vi "Alpha Ver 1.5.vi"() -> ()   [LabVIEW 2015]
uses:
  <instrlib>/Keithley 622x LV 2009/Configure/Source/Typedefs/KE622x -- Current Range.ctl
  <instrlib>/Keithley 622x LV 2009/Configure/Source/Typedefs/KE622x -- Current Ranges.ctl
  <instrlib>/Keithley 622x LV 2009/Typedefs/KE622x -- On Off Control.ctl
  <instrlib>/Keithley 622x LV 2009/Utility/Typedefs/KE622x -- Instrument Type.ctl
  <instrlib>/Keithley 622x LV 2009/Configure/Source/Typedefs/KE622x -- Voltage Limit.ctl
  <instrlib>/Keithley 2000/Public/Configure/Configure DC Volts.vi
  <userlib>/LV-Link3/PolySubVIs/DtCreateAinChan.vi
  <userlib>/LV-Link3/PolySubVIs/DtOLReadMultipleSingle.vi
  <instrlib>/Keithley 2000/Keithley 2000.lvlib
  <instrlib>/Keithley 622x LV 2009/Keithley 622x.lvlib
panel:
  in  "Setup":u16(ring) items=["START, STOP, STEP, CONFIGURATION", "PRINCETON LOCK-IN AMP"]
  out "prev_time_const":i32
  out "prev_range":i32
  out "XTC":i32
  out "SEN":i32
  in  "Time Delay":u16(ring) items=["0.1", "1", "3", "10", "30", "60"]
  out "FILE":refnum<file>
  out "Tick":u32
  in  "MULTIPLE GRAPHS Y":u16(ring) items=["Linear", "Log"]
  in  "MULTIPLE GRAPHS X":u16(ring) items=["Linear", "Log"]
  in  "TIME GRAPH Y":u16(ring) items=["Linear", "Log"]
  in  "TIME GRAPH X":u16(ring) items=["Linear", "Log"]
  in  "Lock-In, Y":dbl=1.0
  in  "Lock-In, X":dbl=1.0
  in  "DAQ A4":dbl=1.0
  in  "DAQ A3":dbl=1.0
  in  "DAQ A2":dbl=1.0
  in  "DAQ A1":dbl=1.0
  in  "DAQ A0":dbl=1.0
  in  "2000":dbl=1.0
  in  "Current":dbl=1000.0
  in  "Display Type 3":u16(ring)=3 items=["X %", "Y %", "X Calibrated", "Y Calibrated", "Mag %", "Mag Calibrated", "Phase Degrees", "Ratio", "ADC 1", "ADC 2", "ADC 3", "ADC 4 ", "Noise %", "Noise Calibrated", "Ref Frequency", "", ""]
  in  "Display Type 2":u16(ring)=2 items=["X %", "Y %", "X Calibrated", "Y Calibrated", "Mag %", "Mag Calibrated", "Phase Degrees", "Ratio", "ADC 1", "ADC 2", "ADC 3", "ADC 4 ", "Noise %", "Noise Calibrated", "Ref Frequency", "", ""]
  out "Units 3":string
  out "Display 3":dbl format="%.3f"
  out "Units 2":string
  out "Display 2":dbl format="%.3f"
  out "DAQ A4":dbl format="%#_13g"
  out "DAQ_clust":T1
  out "DAQ A3":dbl format="%#_13g"
  out "DAQ A2":dbl format="%#_13g"
  out "DAQ A1":dbl format="%#_13g"
  out "Real stop cur":dbl format="%#_13g"
  out "Real start cur":dbl format="%#_13g"
  in  "Stop cur prefix":u16(ring)=2
  in  "Start cur prefix":u16(ring)=2
  out "MULTIPLE GRAPHS":cluster{dbl[], dbl[]}[](graph)
  in  "X-Axis":T2(ring)
  in  "Range":u8(ring)=20 items=["100nV", "200nV", "500nV", "1µV", "2µV", "5µV", "10µV", "20µV", "50µV", "100µV", "200µV", "500µV", "1mV", "2mV", "5mV", "10mV", "20mV", "50mV", "100mV", "200mV", "500mV", "1V"]
  in  "Display Type copy":u16(ring)=3 items=["X %", "Y %", "X Calibrated", "Y Calibrated", "Mag %", "Mag Calibrated", "Phase Degrees", "Ratio", "ADC 1", "ADC 2", "ADC 3", "ADC 4 ", "Noise %", "Noise Calibrated", "Ref Frequency", "", ""]
  out "Units copy":string
  out "Display copy":dbl format="%.3f"
  out "Overload":bool
  out "Display":dbl format="%.3f"
  out "Units":string
  in  "Display Type":u16(ring)=2 items=["X %", "Y %", "X Calibrated", "Y Calibrated", "Mag %", "Mag Calibrated", "Phase Degrees", "Ratio", "ADC 1", "ADC 2", "ADC 3", "ADC 4 ", "Noise %", "Noise Calibrated", "Ref Frequency", "", ""]
  in  "Time Constant":u16(ring)=7 items=["MIN", "1ms", "3ms", "10ms", "30ms", "100ms", "300ms", "1s", "3s", "10s", "30s", "100s", "300s"]
  in  "Slope":u8(ring) items=["6db/octave", "12dB/octave"]
  in  "Dynamic Reserve":u16(ring)=1 items=["High Stability", "Normal", "High Reserve"]
  in  "Auto Sensitivity":bool
  in  "Auto Measure":bool
  out "6221_error_out":errorcluster
  out "2000_error_out":errorcluster
  out "5110_error_out":errorcluster
  out "Input Mode":i32(ring) items=[" Voltage Input (A or A-B) ", "Current Input 10E6 V/A", "Current Input 10E8 V/A"]
  out "5110":refnum<visa-resource-name>
  in  "GPIB Address":i8=11 min=1 max=32 step=1
  out "DAQ A0":dbl format="%#_13g"
  out "2000":dbl format="%#_13g"
  in  "Device":string(combo)
  in  "Number \nof points":i32=10
  in  "Folder\nprename":string
  out "TIME GRAPH":cluster{dbl[], dbl[]}[](graph)
  out "T0":u32
  out "LIMIT":bool
  out "LIMIT":bool
  out "Error Code":string
  in  "Comments":string
  out "2000":refnum<visa-resource-name>
  out "6221":refnum<visa-resource-name>
  out "Step  (A)":dbl=5e-05 format="%#_3p"
  in  "Stop\ncurrent (A)":dbl=2.0 format="%#_6p"
  in  "Start \ncurrent (A)":dbl=1.0 format="%#_6p"
  in  "Check For SCPI Errors? (T)":bool=TRUE
  out "Interlock Tripped?":bool
  out "Compliance?":bool
  in  "Turn Off Output \nIf Compliance?":bool=TRUE
  in  "Turning ON/OFF\ncurrent output":T3=enum."On"
  in  "Range Selection":T4={"Auto Range?"=TRUE, "Man / Selected\nRange"=enum."2nA"}
  # "FILE CONFIGURATION"
  # "ADMIN PANEL"
  # "MULTIPLIERS"
  # "SCALES"
  # "KEITHLEY 6221 CONFIGURATION (ADMIN ONLY)"
  # "KEITHLEY DAQ CONFIGURATION (ADMIN ONLY)"
  # "PRINCETON LOCK-IN AMP (ADMIN ONLY)"
  # "I don't know what the hell it is,\njust don't touch it"
  # "INPUT CONFIGURATION"
  # "READINGS"
  # "IF ON"
  # "Compliance = Limiting output voltage\nThis switch determines if we want to switch \noff the current output if wee exceed compliance"
  # "SCALES"
  # "There is a safe switch at \nthe back of the instrument \nThis indicator shows if it is on"
  # "You have hit a damn jackpot \nby exceeding the limited voltage\nCongrats"
  # "LOCK-IN READINGS"
  # "RIGHT DISPLAY"
  # "LEFT DISPLAY"
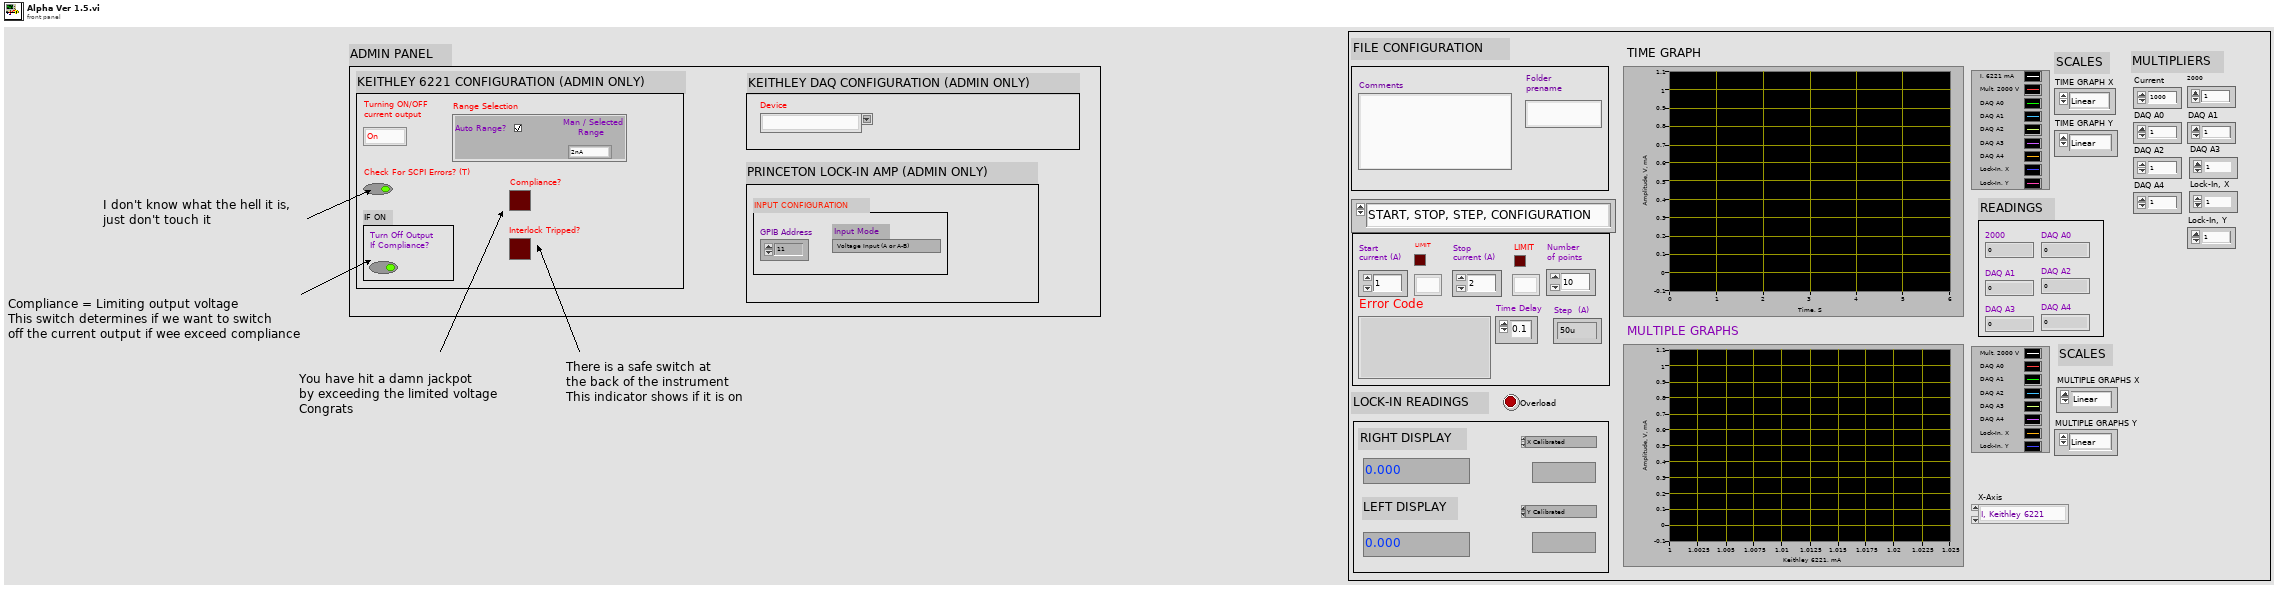
[diagram p1: front panel]
types:
  T1 = cluster{"Task out":i32, "Actual Number of Channels":u32, "error out":errorcluster}
  T2 = enum16{"I, Keithley 6221", "V, Keithley 2000", "V, Keithley DAQ A0", "V, Keithley DAQ A1", "V, Keithley DAQ A2", "V, Keithley DAQ A3", "V, Keithley DAQ A4", "V, Lock-In X", "V, Lock-In Y"}
  T3 = typedef "Keithley 622x.lvlib/KE622x -- On Off Control.ctl" = enum16{"Off", "On"}
  T4 = typedef "Keithley 622x.lvlib/KE622x -- Current Range.ctl" = cluster{"Auto Range?":bool, "Man / Selected\nRange":T5}
  T5 = typedef "Keithley 622x.lvlib/KE622x -- Current Ranges.ctl" = enum16{"2nA", "20nA", "200nA", "2uA", "20uA", "200uA", "2mA", "20mA", "100mA"}
  T6 = typedef "Keithley 622x.lvlib/KE622x -- Instrument Type.ctl" = enum16{"KE6220", "KE6221"}
  T7 = typedef "Keithley 622x.lvlib/KE622x -- Voltage Limit.ctl" = dbl
  T8 = cluster{"Task out":i32, "error out":errorcluster}
  T9 = cluster{dbl, dbl, dbl, dbl, dbl, "Measurement":dbl}
  T10 = cluster{dbl[], dbl[], dbl[], dbl[], dbl[], dbl[], dbl[], dbl[], dbl[], dbl[]}
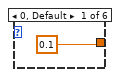
[diagram p2: hidden frame]
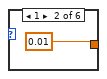
[diagram p3: hidden frame]
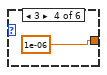
[diagram p4: hidden frame]
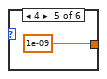
[diagram p5: hidden frame]
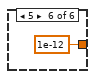
[diagram p6: hidden frame]
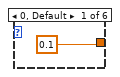
[diagram p7: hidden frame]
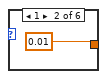
[diagram p8: hidden frame]
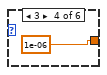
[diagram p9: hidden frame]
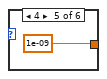
[diagram p10: hidden frame]
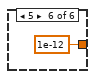
[diagram p11: hidden frame]
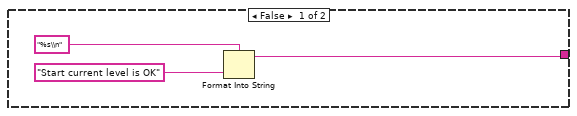
[diagram p12: hidden frame]
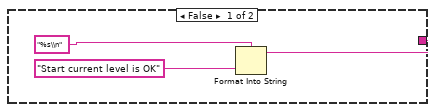
[diagram p13: hidden frame]
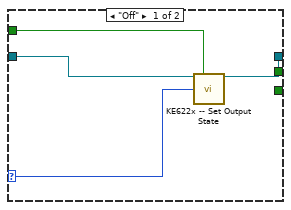
[diagram p14: hidden frame]
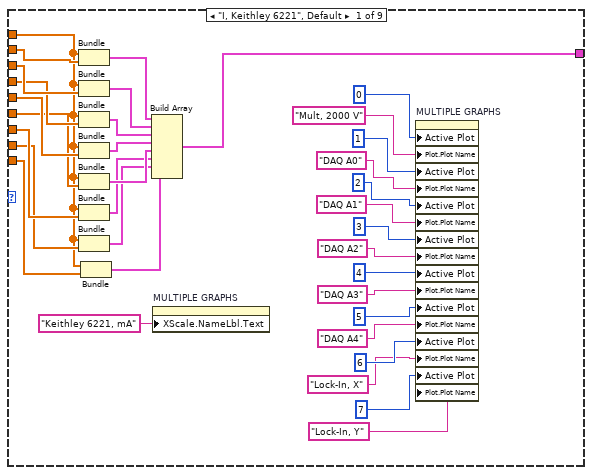
[diagram p15: hidden frame]
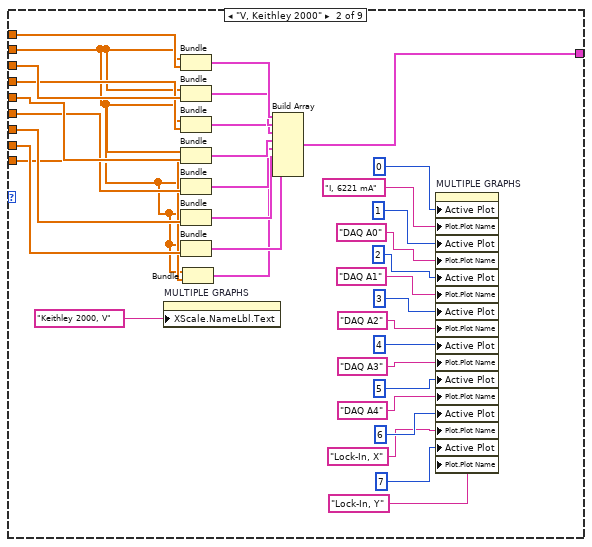
[diagram p16: hidden frame]
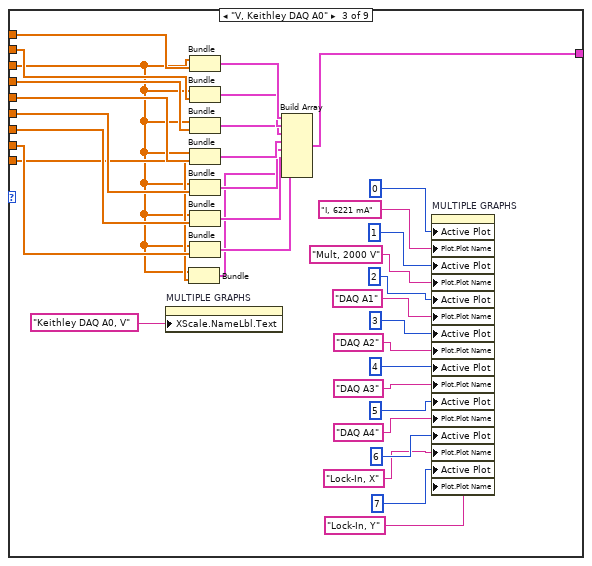
[diagram p17: hidden frame]
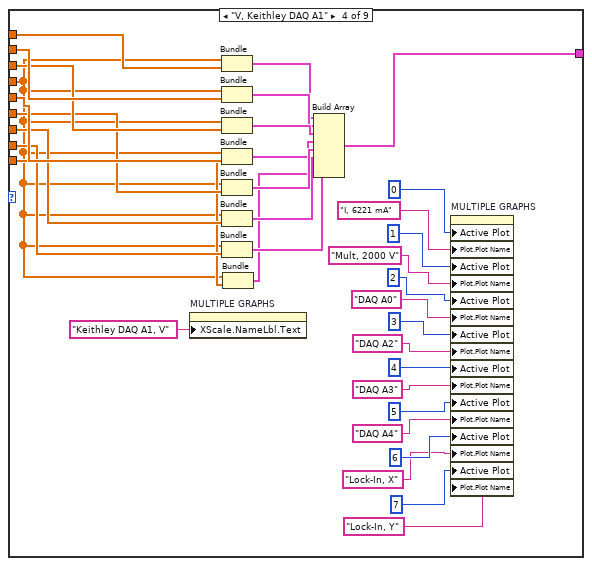
[diagram p18: hidden frame]
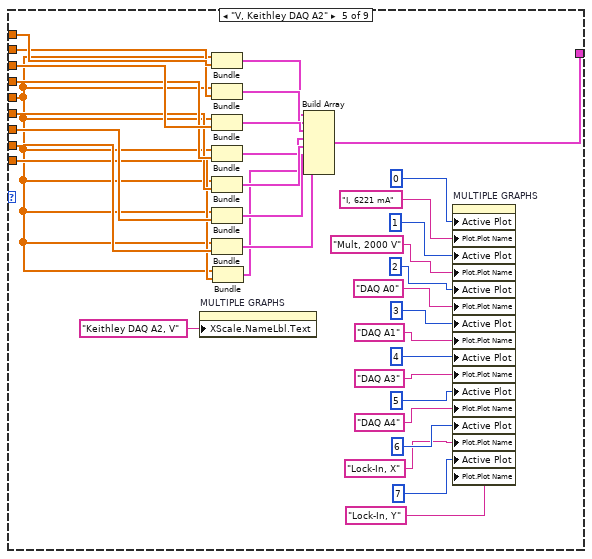
[diagram p19: hidden frame]
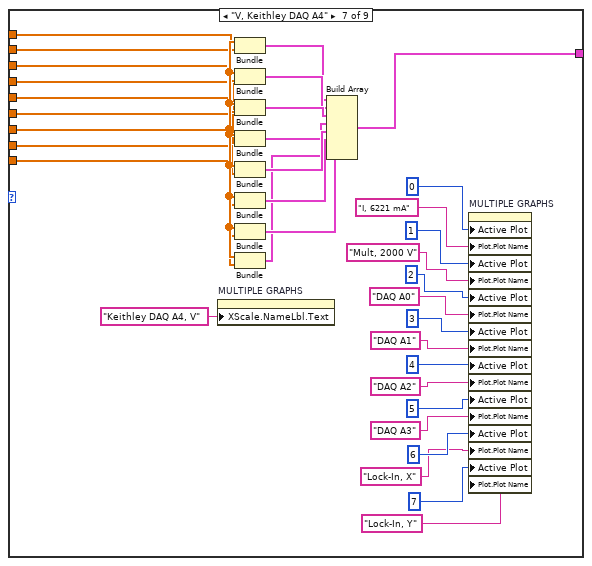
[diagram p20: hidden frame]
diagram:
  n1 = flat-sequence {
    tunnel: [w179] -> w7
    tunnel: [w178] -> w6
    tunnel: [w177] -> w5
    tunnel: [w176] -> w4
    tunnel: [w175] -> w3
    tunnel: [w174] -> w2
    tunnel: [w163] -> w1
    tunnel: w7 -> [w1126]
    tunnel: w6 -> [w1125]
    tunnel: w5 -> [w1124]
    tunnel: w4 -> [w1123]
    tunnel: w3 -> [w1122]
    tunnel: w2 -> [w1121]
    tunnel: w1 -> [w1120]
    frame #0 {
      # "File configuration"
      # "Start, Stop, Step"
      # "Initializing instruments"
      n2 = flat-sequence {
        frame #0 {
          w15 = TRUE  # reset
          w14 = FALSE  # ID query
          # "Initialize Lock-In 5110"
          # "Initialize Keithley 2000"
          # "Initialize Keithley 6221"
          n3 = call <instrlib>:"Initialize.vi"("VISA resource name"=refnum<visa-resource-name> "KEITHLEY_MULTIMETER") -> ("VISA resource name out"=w19:refnum<visa-resource-name>)  [unwired: 17 in, 1 out]
          n4 = call <instrlib>:"Initialize.vi"("VISA resource name"=refnum<visa-resource-name> "KEITHLEY_DC_AC_CURRENT_SOURCE", "Error Queue Option"=enum16{"Clear Error Queue", "Error Query"}."Clear Error Queue", "Instrument Type"=KE622x_--_Instrument_Type."KE6221") -> ("VISA resource name out"=→"6221":refnum<visa-resource-name>, "error out"=→"6221_error_out":errorcluster)  [unwired: 11 in]
          n5 = call "SR51XX Initialize"("VISA session (for class)"=refnum<visa-resource-name> "LOCK_IN_5110_PRINCETON", "Interface"=FALSE, "ID query"=w14, "GPIB Address"="GPIB Address", "reset"=w15) -> ("VISA session"=→"5110":refnum<visa-resource-name>, "error out"=→"5110_error_out":errorcluster)  [unwired: 8 in, 1 out]
          n6 = call-poly <instrlib>:"Configure Measurement.vi"("VISA resource name"=w19) -> ("VISA resource name out"=→"2000":refnum<visa-resource-name>, "error out"=→"2000_error_out":errorcluster)  [unwired: 17 in]
        }
        frame #1 {
          # "Initialize Keithley DAQ \n(getting board name)"
          n7 = call <userlib>:"DtOLGetBoardNames.vi"() -> ("Number of boards"=w24:u32)  [unwired: 9 in, 2 out]
          n8 = Initialize Array("", w24) -> (w26:string[])
          n9 = for {
            N: w24 -> [_]
            shift-right: [w32] -> w29
            shift-left: w26 -> [w33]
            i -> [w31]
            n10 = Add(x=1, y=w31) -> (x+y=w35:i32)
            n11 = call <userlib>:"DtOLGetBoardNames.vi"("Select Board"=w35) -> ("Board Name"=w30:string)  [unwired: 8 in, 2 out]
            n12 = Replace Array Subset(array=w33, new element=w30, index=w31) -> (w32:string[])
          }
          n13 = Index Array(array=w29, index=0) -> (element=w28:string)
          n14 = property on="Device" class="CmbBox"("Strings[]"=w29, "Value"=w28) -> ()  [unwired: 2 in, 2 out]
        }
        frame #2 {
          # "Calculating steps by number\nof points"
          # "Putting in a loop \ninstead of \"STOP\""
          n15 = local read "Real stop cur"() -> (w52:dbl)
          n16 = local read "Real start cur"() -> (w53:dbl)
          n17 = case shown="2" "Start cur prefix" {
            tunnel: [0.1 0.01 0.001 1e-06 1e-09 1e-12] -> w41
            frame 0, Default {
            }
            frame 1 {
            }
            frame 2 {
            }
            frame 3 {
            }
            frame 4 {
            }
            frame 5 {
            }
          }
          n18 = case shown="2" "Stop cur prefix" {
            tunnel: [0.1 0.01 0.001 1e-06 1e-09 1e-12] -> w39
            frame 0, Default {
            }
            frame 1 {
            }
            frame 2 {
            }
            frame 3 {
            }
            frame 4 {
            }
            frame 5 {
            }
          }
          n19 = Subtract(x=w52, y=w53) -> (x-y=w55:dbl)
          n20 = Multiply(x=w41, y="Start \ncurrent (A)") -> (x*y=w37:dbl)
          "Real start cur" <- w37
          n21 = Divide(x=w55, y="Number \nof points") -> (x/y=→"Step  (A)":dbl)
          n22 = Multiply(x=w39, y="Stop\ncurrent (A)") -> (x*y=w36:dbl)
          "Real stop cur" <- w36
          n23 = Greater?(x=w36, y=T7 0.01) -> (0:w47:bool)
          n24 = Greater?(x=w37, y=T7 0.01) -> (0:w46:bool)
          n25 = case shown="True" w47 {
            selector: w47 -> [_ w71]
            tunnel: [w68 w74] -> w49
            frame False {
              n26 = Format Into String(format string="%s\\n", "Start current level is OK" ("false string")) -> (resulting string=w68:string)  [unwired: 2 in, 1 out]
            }
            frame True {
              n27 = flat-sequence {
                tunnel: [w76] -> w73
                tunnel: [w75] -> w72
                tunnel: w71 -> [w75]
                tunnel: [w80] -> w74
                tunnel: w73 -> [w80]
                tunnel: w72 -> [w81]
                frame #0 {
                  n28 = Format Into String(format string="%s\\n%s\\n", "Stop current level" ("String"), "exceeded the  limit: 10mA" ("input 2")) -> (resulting string=w76:string)  [unwired: 2 in, 1 out]
                }
                frame #1 {
                  n29 = while {
                    tunnel: w81 -> [w82]
                    stop <- w82 continue-if-true
                    "LIMIT" <- w82
                  }
                  n30 = property on="Error Code" class="Str"("Text.Text"=w80) -> ()  [unwired: 2 in, 2 out]
                }
              }
            }
          }
          n31 = case shown="True" w46 {
            selector: w46 -> [_ w87]
            tunnel: [w83 w89] -> w48
            frame False {
              n32 = Format Into String(format string="%s\\n", "Start current level is OK" ("false string")) -> (resulting string=w83:string)  [unwired: 2 in, 1 out]
            }
            frame True {
              n33 = flat-sequence {
                tunnel: [w91] -> w88
                tunnel: w87 -> [w90]
                tunnel: [w90] -> w86
                tunnel: [w95] -> w89
                tunnel: w88 -> [w95]
                tunnel: w86 -> [w96]
                frame #0 {
                  n34 = Format Into String(format string="%s\\n%s\\n", "Start current level" ("String"), "exceeded the limit: 10mA" ("input 2")) -> (resulting string=w91:string)  [unwired: 2 in, 1 out]
                }
                frame #1 {
                  n35 = while {
                    tunnel: w96 -> [w97]
                    stop <- w97 continue-if-true
                    "LIMIT" <- w97
                  }
                  n36 = property on="Error Code" class="Str"("Text.Text"=w95) -> ()  [unwired: 2 in, 2 out]
                }
              }
            }
          }
          n37 = Concatenate Strings(w48, w49) -> (→"Error Code":string)
        }
        frame #3 {
          # "Adding headlines"
          # "Creating folder&file"
          # "Creating comments"
          # "Writing instr params"
          n38 = local read "5110"() -> (w110:refnum<visa-resource-name>)
          n39 = local read "Real stop cur"() -> (w112:dbl)
          n40 = local read "Real start cur"() -> (w111:dbl)
          n41 = call "folder_creation.vi"("Name"="Folder\nprename") -> ("String"=w119:string)
          n42 = call "file_creation.vi"("String"=w119) -> ("refnum out"=w113:refnum<file>)
          "FILE" <- w113
          n43 = call "com_inst.vi"("Stop current"=w112, "Start current"=w111, "VISA session (for class)"=w110) -> ("XTC"=w108:i32, "SEN"=w109:i32, "concatenated string"=w107:string)
          "SEN" <- w109
          "XTC" <- w108
          n44 = Format Into String(format string="# %s\\n", initial string=w113, "Comments") -> (resulting string=w115:refnum<file>)  [unwired: 1 in, 1 out]
          n45 = property on="Time Constant" class="Ring (strict)"("Value"=w108) -> ()  [unwired: 2 in, 2 out]
          n46 = Format Into String(format string="# %s\\n", initial string=w115, w107) -> (resulting string=w114:refnum<file>)  [unwired: 1 in, 1 out]
          n47 = property on="Range" class="Ring (strict)"("Value"=w109) -> ()  [unwired: 2 in, 2 out]
          n48 = Format Into String(format string="# %-6s  %-12s %-12s %-14s %-12s %-14s %-12s %-12s %-14s%-14s\\n", initial string=w114, "t, ms" ("input 3"), "6221, A" ("input 3"), "2000, V" ("input 1"), "5110_X, V" ("input 3"), "5110_Y, V " ("input 3"), "DAQ A0, V" ("input 2"), "DAQ A1, V" ("input 2"), "DAQ A2, V" ("input 2"), "DAQ A3, V" ("input 2"), "DAQ A4, V" ("input 2")) -> ()  [unwired: 1 in, 2 out]
        }
        frame #4 {
          # "Variables"
          # "Time Intit"
          n49 = property on="SEN" class="DigNum (strict)"() -> ("Value"=→"prev_range":i32)  [unwired: 2 in, 2 out]
          n50 = property on="XTC" class="DigNum (strict)"() -> ("Value"=→"prev_time_const":i32)  [unwired: 2 in, 2 out]
          n51 = Wait Until Next ms Multiple(millisecond multiple=u32 1000) -> (millisecond timer value=→"T0":u32)
        }
      }
    }
    frame #1 {
      # "Configuring Keithley DAQ just before measuments"
      # "Configuring Keithley 6221 just before measuments"
      n52 = flat-sequence {
        tunnel: [w137] -> w127
        tunnel: [w155] -> _
        tunnel: [w157] -> _
        tunnel: w127 -> [w156]
        frame #0 {
          # "Current range \nselection check"
          # "Checking for compliance\nand interlock errors"
          n53 = local read "6221"() -> (w140:refnum<visa-resource-name>)
          n54 = call <instrlib>:"KE622x -- Set Current Range.vi"("Resource In"=w140, "Current Range In"="Range Selection", "Read Back Set Values? (T)"=FALSE) -> ("Resource Out (dupl)"=w145:refnum<visa-resource-name>)  [unwired: 10 in, 2 out]
          n55 = case shown="\"On\"" "Turning ON/OFF\ncurrent output" {
            selector: "Turning ON/OFF\ncurrent output" -> [w149 _]
            tunnel: [_ w153] -> w143
            tunnel: [_ w152] -> w144
            tunnel: "Check For SCPI Errors? (T)" -> [w148 _]
            tunnel: w145 -> [w146 w151]
            tunnel: [w147 w150] -> w137
            frame "Off" {
              n56 = call <instrlib>:"KE622x -- Set Output State.vi"("Resource In"=w146, "Check For SCPI Errors? (T)"=w148, "Output State"=w149) -> ("Resource Out (dupl)"=w147:refnum<visa-resource-name>)  [unwired: 11 in, 1 out]
            }
            frame "On" {
              n57 = call <instrlib>:"KE622x -- Turn Output On And Check For Errors.vi"("Resource In"=w151, "Turn Off Output If Compliance?"="Turn Off Output \nIf Compliance?") -> ("Resource Out (dupl)"=w150:refnum<visa-resource-name>, "Interlock Tripped?"=w153:bool, "Compliance?"=w152:bool)  [unwired: 10 in, 1 out]
            }
          }
          "Interlock Tripped?" <- w143
          "Compliance?" <- w144
        }
        frame #1 {
          # "Setting start current"
          n58 = local read "Real start cur"() -> (w155:dbl)
          n59 = Wait (ms)(milliseconds to wait=u32 100) -> ()  [unwired: 1 out]
          n60 = call <instrlib>:"KE622x -- Set Current Level.vi"("Resource In"=w156, "Current Level (A) In"=w155) -> ("Resource Out (dupl)"=w157:refnum<visa-resource-name>)  [unwired: 12 in, 1 out]
        }
      }
      n61 = flat-sequence {
        frame #0 {
          w132 = 100 items=["SingleEnded"=100, "Differential"=101] ("Channel Type")
          # "Configure the input channel"
          n62 = call-poly <userlib>:"DtOLCreateTask.vi"("Channel Type"=w132, "Range Min"=-10.0, "Range Max"=10.0, "Board Name"="Device", "Channel"="0:4" ("Channels")) -> ("Task out"=w131:i32, "Actual Number of Channels"=w130:u32, "error out"=w129:errorcluster)  [unwired: 8 in]
          n63 = Bundle("Task out"=w131, "Actual Number of Channels"=w130, "error out"=w129) -> (→"DAQ_clust":T1)  [unwired: 1 in]
        }
      }
    }
    frame #2 {
      n64 = local read "5110"() -> (w170:refnum<visa-resource-name>)
      n65 = local read "2000"() -> (w169:refnum<visa-resource-name>)
      n66 = local read "6221"() -> (w168:refnum<visa-resource-name>)
      n67 = local read "5110_error_out"() -> (w167:errorcluster)
      n68 = local read "6221_error_out"() -> (w166:errorcluster)
      n69 = local read "2000_error_out"() -> (w165:errorcluster)
      n70 = local read "DAQ_clust"() -> (w164:T1)
      n71 = while {
        shift-right: [w380] -> _
        shift-left: dbl[] [] -> [w481]
        shift-right: [w381] -> _
        shift-left: i32[] [] -> [w480]
        tunnel: w169 -> [w478]
        tunnel: w168 -> [w477]
        shift-right: [w338] -> _
        shift-left: dbl[] [] -> [w471]
        tunnel: [w470] -> w179
        tunnel: [w469] -> w178
        tunnel: [w467] -> w177
        tunnel: [w465] -> w176
        tunnel: w170 -> [w463]
        tunnel: w167 -> [w462]
        tunnel: w166 -> [w454]
        tunnel: w165 -> [w453]
        tunnel: [w428] -> w175
        tunnel: [w426] -> w174
        shift-right: [w340] -> _
        shift-left: dbl[] [] -> [w425]
        shift-right: [w341] -> _
        shift-left: dbl[] [] -> [w424]
        shift-right: [w382] -> _
        shift-left: dbl[] [] -> [w421]
        tunnel: w164 -> [w395]
        tunnel: [w394] -> w163
        shift-right: [w379] -> _
        shift-left: dbl[] [] -> [w393]
        shift-right: [w378] -> _
        shift-left: dbl[] [] -> [w392]
        shift-right: [w377] -> _
        shift-left: dbl[] [] -> [w391]
        shift-right: [w339] -> _
        shift-left: dbl[] [] -> [w343]
        i -> [w455]
        stop <- w472 stop-if-true
        # "V, DAQ A4"
        # "V, DAQ A3"
        # "V, DAQ A2"
        # "V, DAQ A1"
        # "Y-V, 5110"
        # "X-V, 5110"
        # "I, 6221"
        # "Config delay"
        # "Control subVI 5110"
        # "Read config 5110"
        # "Measurement config 5110"
        # "Time config 5110"
        # "Configuring Right Display 5110"
        # "Configuring Left Display 5110"
        # "Setting 6221 current"
        # "Delay before measuremens"
        # "Getting the data from DAQ and 2000"
        # "Changing input current"
        # "Time"
        # "V, DAQ A0"
        # "V, 2000"
        n72 = local read "T0"() -> (w479:u32)
        n73 = Quotient & Remainder(x=w455, y=10) -> (floor(x/y)=w460:i32)  [unwired: 1 out]
        n74 = Equal?(x=0, y=w455) -> (x = y?=w457:bool)
        n75 = Subtract(x=w446, y=w479) -> (x-y=w402:u32)
        n76 = Equal?(x=1, y=w460) -> (x = y?=w456:bool)
        n77 = flat-sequence {
          tunnel: w478 -> [w806]
          tunnel: [w806] -> w420
          tunnel: w477 -> [w805]
          tunnel: [w805] -> w418
          tunnel: w463 -> [w804]
          tunnel: [w804] -> w416
          tunnel: [w803] -> w414
          tunnel: w462 -> [w803]
          tunnel: w457 -> [w802]
          tunnel: [w802] -> w412
          tunnel: w456 -> [w801]
          tunnel: [w801] -> w410
          tunnel: w454 -> [w800]
          tunnel: [w800] -> w408
          tunnel: w453 -> [w799]
          tunnel: [w799] -> w406
          tunnel: [w797] -> w446
          tunnel: [w798] -> w396
          tunnel: w395 -> [w798]
          tunnel: w420 -> [w816]
          tunnel: [w816] -> w419
          tunnel: w418 -> [w815]
          tunnel: [w815] -> w417
          tunnel: w416 -> [w814]
          tunnel: [w814] -> w415
          tunnel: w414 -> [w813]
          tunnel: [w813] -> w413
          tunnel: w412 -> [w812]
          tunnel: [w812] -> w411
          tunnel: w410 -> [w811]
          tunnel: [w811] -> w409
          tunnel: w408 -> [w810]
          tunnel: [w810] -> w407
          tunnel: w406 -> [w809]
          tunnel: [w809] -> w405
          tunnel: [w808] -> w397
          tunnel: w396 -> [w808]
          tunnel: w419 -> [w861]
          tunnel: [w861] -> w445
          tunnel: w417 -> [w860]
          tunnel: [w860] -> w444
          tunnel: w415 -> [w859]
          tunnel: w413 -> [w856]
          tunnel: [w855] -> w443
          tunnel: [w854] -> w442
          tunnel: w411 -> [w853]
          tunnel: [w853] -> w441
          tunnel: w409 -> [w852]
          tunnel: w407 -> [w851]
          tunnel: [w851] -> w440
          tunnel: w405 -> [w850]
          tunnel: [w850] -> w439
          tunnel: [w849] -> w398
          tunnel: w397 -> [w849]
          tunnel: w445 -> [w886]
          tunnel: [w886] -> w239
          tunnel: w444 -> [w885]
          tunnel: [w885] -> w237
          tunnel: w443 -> [w882]
          tunnel: [w881] -> w235
          tunnel: w442 -> [w880]
          tunnel: [w879] -> w233
          tunnel: w441 -> [w877]
          tunnel: [w877] -> w231
          tunnel: w440 -> [w884]
          tunnel: [w884] -> w229
          tunnel: w439 -> [w883]
          tunnel: [w883] -> w227
          tunnel: ["Auto Measure"] -> w225
          tunnel: ["Auto Sensitivity"] -> w223
          tunnel: [w872] -> w221
          tunnel: [w870] -> w219
          tunnel: w398 -> [w870]
          tunnel: w239 -> [w900]
          tunnel: [w900] -> w238
          tunnel: w237 -> [w899]
          tunnel: [w899] -> w236
          tunnel: w235 -> [w887]
          tunnel: [w887] -> w234
          tunnel: w233 -> [w898]
          tunnel: [w898] -> w232
          tunnel: w231 -> [w897]
          tunnel: [w897] -> w230
          tunnel: w229 -> [w896]
          tunnel: [w896] -> w228
          tunnel: w227 -> [w895]
          tunnel: [w895] -> w226
          tunnel: w225 -> [w894]
          tunnel: [w894] -> w224
          tunnel: w223 -> [w893]
          tunnel: [w893] -> w222
          tunnel: w221 -> [w892]
          tunnel: [w892] -> w220
          tunnel: w219 -> [w891]
          tunnel: [w891] -> w218
          tunnel: w238 -> [w927]
          tunnel: [w927] -> w195
          tunnel: w236 -> [w926]
          tunnel: [w926] -> w197
          tunnel: w234 -> [w919]
          tunnel: w232 -> [w917]
          tunnel: [w916] -> w199
          tunnel: w230 -> [w923]
          tunnel: [w923] -> w201
          tunnel: w228 -> [w925]
          tunnel: [w925] -> w203
          tunnel: w226 -> [w924]
          tunnel: [w924] -> w205
          tunnel: w224 -> [w921]
          tunnel: [w921] -> w207
          tunnel: w222 -> [w922]
          tunnel: [w922] -> w209
          tunnel: w220 -> [w912]
          tunnel: [w912] -> w211
          tunnel: [w918] -> w213
          tunnel: ["Time Constant"] -> w215
          tunnel: ["Slope"] -> w217
          tunnel: [w910] -> w193
          tunnel: w218 -> [w910]
          tunnel: w217 -> [w943]
          tunnel: [w943] -> w216
          tunnel: w215 -> [w942]
          tunnel: [w942] -> w214
          tunnel: w213 -> [w930]
          tunnel: [w930] -> w212
          tunnel: w211 -> [w941]
          tunnel: [w941] -> w210
          tunnel: w209 -> [w940]
          tunnel: [w940] -> w208
          tunnel: w207 -> [w939]
          tunnel: [w939] -> w206
          tunnel: w205 -> [w938]
          tunnel: [w938] -> w204
          tunnel: w203 -> [w937]
          tunnel: [w937] -> w202
          tunnel: w201 -> [w936]
          tunnel: [w936] -> w200
          tunnel: w199 -> [w932]
          tunnel: [w932] -> w198
          tunnel: w197 -> [w935]
          tunnel: [w935] -> w196
          tunnel: w195 -> [w934]
          tunnel: [w934] -> w194
          tunnel: w193 -> [w933]
          tunnel: [w933] -> w192
          tunnel: [w973] -> w336
          tunnel: [w972] -> w335
          tunnel: [w958] -> w334
          tunnel: [w971] -> w333
          tunnel: [w970] -> w332
          tunnel: [w969] -> w331
          tunnel: [w968] -> w330
          tunnel: [w967] -> w329
          tunnel: [w960] -> w328
          tunnel: [w963] -> w327
          tunnel: [w961] -> w326
          tunnel: [w966] -> w325
          tunnel: w216 -> [w966]
          tunnel: w214 -> [w961]
          tunnel: w212 -> [w964]
          tunnel: w210 -> [w960]
          tunnel: w208 -> [w967]
          tunnel: w206 -> [w968]
          tunnel: w204 -> [w969]
          tunnel: w202 -> [w970]
          tunnel: w200 -> [w971]
          tunnel: w198 -> [w959]
          tunnel: w196 -> [w972]
          tunnel: w194 -> [w973]
          tunnel: [w952] -> w324
          tunnel: w192 -> [w952]
          tunnel: w336 -> [w996]
          tunnel: [w996] -> w323
          tunnel: w335 -> [w995]
          tunnel: [w995] -> w321
          tunnel: w334 -> [w987]
          tunnel: [w986] -> w319
          tunnel: w333 -> [w994]
          tunnel: [w994] -> w317
          tunnel: w332 -> [w993]
          tunnel: [w993] -> w315
          tunnel: w331 -> [w992]
          tunnel: [w992] -> w313
          tunnel: w330 -> [w991]
          tunnel: [w991] -> w311
          tunnel: w329 -> [w990]
          tunnel: [w990] -> w309
          tunnel: w328 -> [w981]
          tunnel: [w981] -> w307
          tunnel: w327 -> [w988]
          tunnel: [w985] -> w305
          tunnel: w326 -> [w983]
          tunnel: [w983] -> w303
          tunnel: w325 -> [w980]
          tunnel: [w980] -> w301
          tunnel: w324 -> [w989]
          tunnel: [w989] -> w299
          tunnel: [w976] -> w296
          tunnel: w323 -> [w1019]
          tunnel: [w1019] -> w322
          tunnel: w321 -> [w1018]
          tunnel: [w1018] -> w320
          tunnel: w319 -> [w1009]
          tunnel: [w1008] -> w318
          tunnel: w317 -> [w1017]
          tunnel: [w1017] -> w316
          tunnel: w315 -> [w1016]
          tunnel: [w1016] -> w314
          tunnel: w313 -> [w1015]
          tunnel: [w1015] -> w312
          tunnel: w311 -> [w1014]
          tunnel: [w1014] -> w310
          tunnel: w309 -> [w1013]
          tunnel: [w1013] -> w308
          tunnel: w307 -> [w1004]
          tunnel: [w1004] -> w306
          tunnel: w305 -> [w1011]
          tunnel: [w1010] -> w304
          tunnel: w303 -> [w1006]
          tunnel: [w1006] -> w302
          tunnel: w301 -> [w1003]
          tunnel: [w1003] -> w300
          tunnel: w299 -> [w1012]
          tunnel: [w1012] -> w298
          tunnel: [w999] -> w297
          tunnel: w322 -> [w1041]
          tunnel: [w1041] -> w438
          tunnel: w320 -> [w1040]
          tunnel: [w1040] -> w437
          tunnel: w318 -> [w1027]
          tunnel: w316 -> [w1039]
          tunnel: [w1039] -> w436
          tunnel: w314 -> [w1038]
          tunnel: [w1038] -> w435
          tunnel: w312 -> [w1037]
          tunnel: [w1037] -> w434
          tunnel: w310 -> [w1036]
          tunnel: [w1036] -> w433
          tunnel: w308 -> [w1035]
          tunnel: [w1035] -> w432
          tunnel: w306 -> [w1028]
          tunnel: w304 -> [w1025]
          tunnel: [w1024] -> w431
          tunnel: w302 -> [w1029]
          tunnel: w300 -> [w1030]
          tunnel: [w1026] -> w430
          tunnel: [w1023] -> w429
          tunnel: [w1020] -> w399
          tunnel: w298 -> [w1020]
          tunnel: [w1045] -> w476
          tunnel: w455 -> [w1053]
          tunnel: [w1049] -> w472
          tunnel: [w1043] -> w474
          tunnel: [w1051] -> w473
          tunnel: [w1048] -> w452
          tunnel: [w1047] -> w451
          tunnel: [w1046] -> w450
          tunnel: [w1044] -> w449
          tunnel: [w1043] -> w390
          tunnel: w429 -> [_]
          tunnel: w430 -> [w1046]
          tunnel: w431 -> [w1044]
          tunnel: w432 -> [_]
          tunnel: w433 -> [_]
          tunnel: w434 -> [w1048]
          tunnel: w435 -> [w1047]
          tunnel: w436 -> [_]
          tunnel: w437 -> [w1051]
          tunnel: w438 -> [w1045]
          tunnel: [w1042] -> w400
          tunnel: w399 -> [w1042]
          tunnel: w476 -> [w1066]
          tunnel: [w1066] -> w475
          tunnel: w474 -> [w1065]
          tunnel: w473 -> [w1064]
          tunnel: [w1063] -> w468
          tunnel: [w1062] -> w466
          tunnel: w452 -> [w1060]
          tunnel: w451 -> [w1061]
          tunnel: w450 -> [w1058]
          tunnel: w449 -> [w1059]
          tunnel: [w1060] -> w448
          tunnel: [w1059] -> w447
          tunnel: [w1058] -> w427
          tunnel: [w1057] -> w401
          tunnel: w400 -> [w1057]
          tunnel: [w1103] -> w365
          tunnel: [w1070] -> w364
          tunnel: [w1102] -> w363
          tunnel: [w1101] -> w362
          tunnel: [w1100] -> w361
          tunnel: [w1099] -> w360
          tunnel: [w1071] -> w359
          tunnel: [w1103] -> w358
          tunnel: [w1098] -> w357
          tunnel: [w1097] -> w356
          tunnel: [w1096] -> w355
          tunnel: [w1069] -> w354
          tunnel: [w1068] -> w353
          tunnel: [w1067] -> w352
          tunnel: w401 -> [w1093]
          tunnel: w427 -> [w1097]
          tunnel: w447 -> [w1098]
          tunnel: w448 -> [w1094]
          tunnel: w466 -> [w1099]
          tunnel: w468 -> [w1100]
          tunnel: w475 -> [w1095]
          tunnel: [w1107] -> w394
          tunnel: [w1108] -> w426
          tunnel: [w1109] -> w428
          tunnel: [w1110] -> w464
          tunnel: [w1111] -> w351
          tunnel: [w1112] -> w465
          tunnel: [w1113] -> w467
          tunnel: [w1114] -> w469
          tunnel: [w1115] -> w470
          tunnel: [w1116] -> w350
          tunnel: [w1117] -> w346
          tunnel: w365 -> [w1117]
          tunnel: w364 -> [w1116]
          tunnel: w363 -> [w1115]
          tunnel: w362 -> [w1114]
          tunnel: w361 -> [w1113]
          tunnel: w360 -> [w1112]
          tunnel: w359 -> [w1111]
          tunnel: w358 -> [w1110]
          tunnel: w357 -> [w1109]
          tunnel: w356 -> [w1108]
          tunnel: w355 -> [w1107]
          tunnel: [w1106] -> w349
          tunnel: w354 -> [w1106]
          tunnel: [w1105] -> w348
          tunnel: w353 -> [w1105]
          tunnel: w352 -> [w1104]
          tunnel: [w1104] -> w347
          frame #0 {
            n78 = Tick Count (ms)() -> (millisecond timer value=w797:u32)
            "Tick" <- w797
          }
          frame #1 {
            n79 = case shown="0, Default" "Setup" {
              frame 0, Default {
                n80 = property on="Slope" class="Ring (strict)"("Visible"=FALSE) -> ()  [unwired: 2 in, 2 out]
                n81 = property on="Start \ncurrent (A)" class="DigNum (strict)"("Visible"=TRUE) -> ()  [unwired: 2 in, 2 out]
                n82 = property on="LIMIT" class="Bool (strict)"("Visible"=TRUE) -> ()  [unwired: 2 in, 2 out]
                n83 = property on="Start cur prefix" class="Ring (strict)"("Visible"=TRUE) -> ()  [unwired: 2 in, 2 out]
                n84 = property on="Step  (A)" class="DigNum (strict)"("Visible"=TRUE) -> ()  [unwired: 2 in, 2 out]
                n85 = property on="Dynamic Reserve" class="Ring (strict)"("Visible"=FALSE) -> ()  [unwired: 2 in, 2 out]
                n86 = property on="Range" class="Ring (strict)"("Visible"=FALSE) -> ()  [unwired: 2 in, 2 out]
                n87 = property on="LIMIT" class="Bool (strict)"("Visible"=TRUE) -> ()  [unwired: 2 in, 2 out]
                n88 = property on="Stop\ncurrent (A)" class="DigNum (strict)"("Visible"=TRUE) -> ()  [unwired: 2 in, 2 out]
                n89 = property on="Stop cur prefix" class="Ring (strict)"("Visible"=TRUE) -> ()  [unwired: 2 in, 2 out]
                n90 = property on="Time Delay" class="Ring (strict)"("Visible"=TRUE) -> ()  [unwired: 2 in, 2 out]
                n91 = property on="Auto Sensitivity" class="Bool (strict)"("Visible"=FALSE) -> ()  [unwired: 2 in, 2 out]
                n92 = property on="Time Constant" class="Ring (strict)"("Visible"=FALSE) -> ()  [unwired: 2 in, 2 out]
                n93 = property on="Number \nof points" class="DigNum (strict)"("Visible"=TRUE) -> ()  [unwired: 2 in, 2 out]
                n94 = property on="Auto Measure" class="Bool (strict)"("Visible"=FALSE) -> ()  [unwired: 2 in, 2 out]
                n95 = property on="Error Code" class="Str"("Visible"=TRUE) -> ()  [unwired: 2 in, 2 out]
              }
              frame 1 {
                n96 = property on="Slope" class="Ring (strict)"("Visible"=TRUE) -> ()  [unwired: 2 in, 2 out]
                n97 = property on="Start \ncurrent (A)" class="DigNum (strict)"("Visible"=FALSE) -> ()  [unwired: 2 in, 2 out]
                n98 = property on="LIMIT" class="Bool (strict)"("Visible"=FALSE) -> ()  [unwired: 2 in, 2 out]
                n99 = property on="Start cur prefix" class="Ring (strict)"("Visible"=FALSE) -> ()  [unwired: 2 in, 2 out]
                n100 = property on="Step  (A)" class="DigNum (strict)"("Visible"=FALSE) -> ()  [unwired: 2 in, 2 out]
                n101 = property on="Dynamic Reserve" class="Ring (strict)"("Visible"=TRUE) -> ()  [unwired: 2 in, 2 out]
                n102 = property on="Range" class="Ring (strict)"("Visible"=TRUE) -> ()  [unwired: 2 in, 2 out]
                n103 = property on="LIMIT" class="Bool (strict)"("Visible"=FALSE) -> ()  [unwired: 2 in, 2 out]
                n104 = property on="Stop\ncurrent (A)" class="DigNum (strict)"("Visible"=FALSE) -> ()  [unwired: 2 in, 2 out]
                n105 = property on="Time Delay" class="Ring (strict)"("Visible"=FALSE) -> ()  [unwired: 2 in, 2 out]
                n106 = property on="Stop cur prefix" class="Ring (strict)"("Visible"=FALSE) -> ()  [unwired: 2 in, 2 out]
                n107 = property on="Auto Sensitivity" class="Bool (strict)"("Visible"=TRUE) -> ()  [unwired: 2 in, 2 out]
                n108 = property on="Time Constant" class="Ring (strict)"("Visible"=TRUE) -> ()  [unwired: 2 in, 2 out]
                n109 = property on="Auto Measure" class="Bool (strict)"("Visible"=TRUE) -> ()  [unwired: 2 in, 2 out]
                n110 = property on="Number \nof points" class="DigNum (strict)"("Visible"=FALSE) -> ()  [unwired: 2 in, 2 out]
                n111 = property on="Error Code" class="Str"("Visible"=FALSE) -> ()  [unwired: 2 in, 2 out]
              }
            }
          }
          frame #2 {
            n112 = case shown="False" w852 {
              tunnel: w859 -> [w863 w868]
              tunnel: [w862 w866] -> w858
              tunnel: [w863 w865] -> w857
              tunnel: w856 -> [w862 w864]
              frame False {
              }
              frame True {
                n113 = call "SR51XX Read Preamp Input Mode"("VISA session (for class)"=w868, "error in (no error)"=w864) -> ("VISA session"=w865:refnum<visa-resource-name>, "Input Mode"=w867:i32, "error out"=w866:errorcluster)  [unwired: 15 in]
                n114 = local write "Input Mode"(w867) -> ()
              }
            }
            n115 = call "SR51XX Configure Signal Channel Input"("VISA session (for class)"=w857, "error in (no error)"=w858, "Update"=w853) -> ("VISA session"=w855:refnum<visa-resource-name>, "error out"=w854:errorcluster)  [unwired: 15 in]
          }
          frame #3 {
            n116 = local read "Input Mode"() -> (w878:i32)
            n117 = call "SR51XX Configure Sensitivity"("VISA session (for class)"=w882, "Input Mode"=w878, "Range"="Range", "error in (no error)"=w880, "Auto Sensitivity"="Auto Sensitivity", "Auto Measure"="Auto Measure", "Update"=w877) -> ("Range Annotations Out[]"=w871:string[], "VISA session"=w881:refnum<visa-resource-name>, "Auto Sensitivity out"=w874:bool, "Auto Measure out"=w873:bool, "Range Out"=w872:u8, "error out"=w879:errorcluster)  [unwired: 7 in]
            n118 = property on="Range" class="Ring (strict)"("Strings []"=w871) -> ()  [unwired: 2 in, 2 out]
            n119 = local write "Auto Sensitivity"(w874) -> ()
            n120 = local write "Auto Measure"(w873) -> ()
            n121 = local write "Range"(w872) -> ()
          }
          frame #4 {
            n122 = property on="prev_range" class="DigNum (strict)"() -> ("Value"=w889:i32)  [unwired: 2 in, 2 out]
            n123 = property on="Range" class="Ring (strict)"() -> ("Value"=w888:u8)  [unwired: 2 in, 2 out]
            n124 = Equal?(x=w888, y=w889) -> (x = y?=w890:bool)
            n125 = case shown="False" w890 {
              tunnel: w887 -> [w901 _]
              frame False {
                n126 = flat-sequence {
                  tunnel: w901 -> [w903]
                  frame #0 {
                    n127 = property on="Range" class="Ring (strict)"() -> ("Value"=w902:u8)  [unwired: 2 in, 2 out]
                    n128 = property on="prev_range" class="DigNum (strict)"("Value"=w902) -> ()  [unwired: 2 in, 2 out]
                  }
                  frame #1 {
                    n129 = call "read_sense.vi"("VISA session (for class)"=w903) -> ("sense"=w905:string)
                    n130 = Concatenate Strings("Sensitivity: " ("string"), w905) -> (w904:string)
                    n131 = local read "FILE"() -> (w908:refnum<file>)
                    n132 = Format Into String(format string="# %-s\\n", initial string=w908, w904) -> ()  [unwired: 1 in, 2 out]
                  }
                }
              }
              frame True {
              }
            }
          }
          frame #5 {
            n133 = Or(x=w922, y=w921) -> (x .or. y?=w920:bool)
            n134 = call "SR51XX Configure Output Channels - Slope, TC and Dyn Reserve"("VISA session (for class)"=w919, "Time Constant"="Time Constant", "Slope"="Slope", "Check TC"=w920, "Dynamic Reserve"="Dynamic Reserve", "error in (no error)"=w917, "Range"=w912, "Update"=w923) -> ("VISA session"=w918:refnum<visa-resource-name>, "Slope Out"=w913:u8, "Time Constant Out"=w914:u16, "error out"=w916:errorcluster)  [unwired: 8 in]
            n135 = local write "Slope"(w913) -> ()
            n136 = local write "Time Constant"(w914) -> ()
          }
          frame #6 {
            n137 = property on="prev_time_const" class="DigNum (strict)"() -> ("Value"=w929:i32)  [unwired: 2 in, 2 out]
            n138 = property on="Time Constant" class="Ring (strict)"() -> ("Value"=w928:u16)  [unwired: 2 in, 2 out]
            n139 = Equal?(x=w928, y=w929) -> (x = y?=w931:bool)
            n140 = case shown="False" w931 {
              tunnel: w930 -> [w944 _]
              frame False {
                n141 = flat-sequence {
                  tunnel: w944 -> [w946]
                  frame #0 {
                    n142 = property on="Time Constant" class="Ring (strict)"() -> ("Value"=w945:u16)  [unwired: 2 in, 2 out]
                    n143 = property on="prev_time_const" class="DigNum (strict)"("Value"=w945) -> ()  [unwired: 2 in, 2 out]
                  }
                  frame #1 {
                    n144 = call "read_time_const.vi"("VISA session (for class)"=w946) -> ("time_const"=w947:string)
                    n145 = Concatenate Strings("Time Constant: " ("string"), w947) -> (w948:string)
                    n146 = local read "FILE"() -> (w951:refnum<file>)
                    n147 = Format Into String(format string="# %-s\\n", initial string=w951, w948) -> ()  [unwired: 1 in, 2 out]
                  }
                }
              }
              frame True {
              }
            }
          }
          frame #7 {
            n148 = local read "Input Mode"() -> (w965:i32)
            n149 = call "SR5110 Read Output"("VISA session (for class)"=w964, "Input Mode"=w965, "Time Constant"=w961, "Display Type"="Display Type", "Range"=w960, "error in (no error)"=w959, "Slope"=w966) -> ("Units"=→"Units":string, "Display Precision"=w957:i32, "Display"=→"Display":dbl, "VISA session"=w963:refnum<visa-resource-name>, "Available Display Types Out"=w956:string[], "Overload"=→"Overload":bool, "error out"=w958:errorcluster)  [unwired: 4 in, 2 out]
            n150 = property on="Display Type" class="Ring (strict)"("Strings []"=w956) -> ()  [unwired: 2 in, 2 out]
            n151 = property on="Display" class="DigNum (strict)"("Precision"=w957) -> ()  [unwired: 2 in, 2 out]
          }
          frame #8 {
            n152 = local read "Input Mode"() -> (w984:i32)
            n153 = call "SR5110 Read Output"("VISA session (for class)"=w988, "Input Mode"=w984, "Time Constant"=w983, "Display Type"="Display Type 2", "Range"=w981, "error in (no error)"=w987, "Slope"=w980) -> ("Units"=w974:string, "Display Precision"=w978:i32, "Display"=w975:dbl, "VISA session"=w985:refnum<visa-resource-name>, "Available Display Types Out"=w979:string[], "error out"=w986:errorcluster)  [unwired: 4 in, 3 out]
            "Display 2" <- w975
            "Units 2" <- w974
            n154 = call "pref_to_num.vi"("string"=w974) -> ("Numeric"=w977:dbl)
            n155 = property on="Display Type 2" class="Ring (strict)"("Strings []"=w979) -> ()  [unwired: 2 in, 2 out]
            n156 = property on="Display 2" class="DigNum (strict)"("Precision"=w978) -> ()  [unwired: 2 in, 2 out]
            n157 = Multiply(x=w977, y=w975) -> (x*y=w976:dbl)
          }
          frame #9 {
            n158 = local read "Input Mode"() -> (w1007:i32)
            n159 = call "SR5110 Read Output"("VISA session (for class)"=w1011, "Input Mode"=w1007, "Time Constant"=w1006, "Display Type"="Display Type 3", "Range"=w1004, "error in (no error)"=w1009, "Slope"=w1003) -> ("Units"=w998:string, "Display Precision"=w1002:i32, "Display"=w997:dbl, "VISA session"=w1010:refnum<visa-resource-name>, "Available Display Types Out"=w1001:string[], "error out"=w1008:errorcluster)  [unwired: 4 in, 3 out]
            "Display 3" <- w997
            "Units 3" <- w998
            n160 = property on="Display 3" class="DigNum (strict)"("Precision"=w1002) -> ()  [unwired: 2 in, 2 out]
            n161 = call "pref_to_num.vi"("string"=w998) -> ("Numeric"=w1000:dbl)
            n162 = property on="Display Type 3" class="Ring (strict)"("Strings []"=w1001) -> ()  [unwired: 2 in, 2 out]
            n163 = Multiply(x=w1000, y=w997) -> (x*y=w999:dbl)
          }
          frame #10 {
            n164 = local read "Input Mode"() -> (w1034:i32)
            n165 = call "SR5110 Read Output"("VISA session (for class)"=w1025, "Input Mode"=w1034, "Time Constant"=w1029, "Display Type"="Display Type copy", "Range"=w1028, "error in (no error)"=w1027, "Slope"=w1030) -> ("Units"=→"Units copy":string, "Display Precision"=w1031:i32, "Display"=→"Display copy":dbl, "VISA session"=w1024:refnum<visa-resource-name>, "Reference Unlock"=w1023:bool, "Available Display Types Out"=w1032:string[], "error out"=w1026:errorcluster)  [unwired: 4 in, 2 out]
            n166 = property on="Display Type copy" class="Ring (strict)"("Strings []"=w1032) -> ()  [unwired: 2 in, 2 out]
            n167 = property on="Display copy" class="DigNum (strict)"("Precision"=w1031) -> ()  [unwired: 2 in, 2 out]
          }
          frame #11 {
            n168 = local read "Step  (A)"() -> (w1054:dbl)
            n169 = local read "Real start cur"() -> (w1055:dbl)
            n170 = Multiply(x=w1054, y=w1053) -> (x*y=w1052:dbl)
            n171 = Add(x=w1055, y=w1052) -> (x+y=w1043:dbl)
            n172 = local read "Real stop cur"() -> (w1050:dbl)
            n173 = Greater Or Equal?(x=w1043, y=w1050) -> (x >= y?=w1049:bool)
          }
          frame #12 {
            n174 = call <instrlib>:"KE622x -- Set Current Level.vi"("Resource In"=w1064, "Current Level (A) In"=w1065, "error in (no error)"=w1061) -> ("Resource Out (dupl)"=w1062:refnum<visa-resource-name>, "error out"=w1063:errorcluster)  [unwired: 11 in]
            n175 = Wait Until Next ms Multiple(millisecond multiple=u32 50) -> ()  [unwired: 1 out]
          }
          frame #13 {
            n176 = Unbundle(w1093) -> ("Task out"=w1092:i32, "Actual Number of Channels"=w1090:u32, "error out"=w1091:errorcluster)
            n177 = call <instrlib>:"Data Read Single.vi"("VISA resource name"=w1095, "error in (no error)"=w1094) -> ("VISA resource name out"=w1101:refnum<visa-resource-name>, "Measurement"=w1103:dbl, "error out"=w1102:errorcluster)  [unwired: 13 in, 2 out]
            n178 = call-poly <userlib>:"DtOLRead.vi"("Number Chan to Read"=w1090, "error in (no error)"=w1091, "Task in"=w1092) -> ("error out"=w1088:errorcluster, "2D Data out"=w1087:dbl[][], "Task out"=w1089:i32)  [unwired: 4 in, 2 out]
            n179 = Index Array(array=w1087, index (row) #1=0 ("index (row)"), index (row) #2=1 ("index (row)"), index (row) #3=2 ("index (row)"), index (row) #4=3 ("index (row)"), index (row) #5=4 ("index (row)")) -> (element #1=w1086:dbl[], element #2=w1080:dbl[], element #3=w1079:dbl[], element #4=w1078:dbl[], element #5=w1077:dbl[])  [unwired: 5 in]
            n180 = Index Array(array=w1077, index=0) -> (element=w1067:dbl)
            n181 = Index Array(array=w1086, index=0) -> (element=w1071:dbl)
            n182 = Index Array(array=w1080, index=0) -> (element=w1070:dbl)
            n183 = Index Array(array=w1079, index=0) -> (element=w1069:dbl)
            n184 = Index Array(array=w1078, index=0) -> (element=w1068:dbl)
            n185 = Bundle("Task out"=w1089, "error out"=w1088) -> (w1096:T8)  [unwired: 1 in]
          }
          frame #14 {
          }
        }
        n186 = Divide(x=w402, y=u32 1000) -> (x/y=w403:dbl)
        n187 = local read "FILE"() -> (w243:refnum<file>)
        n188 = Build Array (concatenate)(w480, w403) -> (w388:dbl[])
        n189 = property on="TIME GRAPH" class="XYGraph (strict)"("XScale.Mapping Mode"="TIME GRAPH X", "YScale.Mapping Mode"="TIME GRAPH Y") -> ()  [unwired: 2 in, 2 out]
        n190 = property on="MULTIPLE GRAPHS" class="XYGraph (strict)"("XScale.Mapping Mode"="MULTIPLE GRAPHS X", "YScale.Mapping Mode"="MULTIPLE GRAPHS Y") -> ()  [unwired: 2 in, 2 out]
        n191 = Bundle(w390, w296, w297) -> (w249:cluster{dbl, dbl, dbl})  [unwired: 1 in]
        n192 = Unbundle(w249) -> (w293:dbl, w259:dbl, w254:dbl)
        n193 = Unbundle(w249) -> (w191:dbl, w190:dbl, w189:dbl)
        n194 = Multiply(x=w293, y="Current") -> (x*y=w292:dbl)
        n195 = Multiply(x=w254, y="Lock-In, Y") -> (x*y=w255:dbl)
        n196 = Multiply(x=w259, y="Lock-In, X") -> (x*y=w260:dbl)
        n197 = Build Array (concatenate)(w421, w292) -> (w389:dbl[])
        n198 = Build Array (concatenate)(w425, w260) -> (w345:dbl[])
        n199 = Build Array (concatenate)(w424, w255) -> (w344:dbl[])
        n200 = Bundle(w351, w350, w349, w348, w347, "Measurement"=w346) -> (w366:T9)  [unwired: 1 in]
        n201 = Unbundle(w366) -> (w285:dbl, w279:dbl, w274:dbl, w269:dbl, w264:dbl, "Measurement"=w288:dbl)
        n202 = Unbundle(w366) -> (w187:dbl, w186:dbl, w185:dbl, w184:dbl, w183:dbl, "Measurement"=w188:dbl)
        n203 = Format Into String(format string="%08d  %8.2e %12g %14.5e %12.4e %12.4e  %12.4e %12.4e  %12.4e  %12g \\n", initial string=w243, w402, w191, w188, w190, w189, w187, w186, w185, w184, w183) -> ()  [unwired: 1 in, 2 out]
        n204 = Multiply(x=w288, y="2000") -> (x*y=w286:dbl)
        n205 = Multiply(x=w279, y="DAQ A1") -> (x*y=w280:dbl)
        n206 = Multiply(x=w285, y="DAQ A0") -> (x*y=w284:dbl)
        n207 = Multiply(x="DAQ A2", y=w274) -> (x*y=w275:dbl)
        n208 = Multiply(x=w264, y="DAQ A4") -> (x*y=w265:dbl)
        n209 = Multiply(x=w269, y="DAQ A3") -> (x*y=w270:dbl)
        n210 = Build Array (concatenate)(w481, w286) -> (w387:dbl[])
        n211 = Build Array (concatenate)(w393, w284) -> (w386:dbl[])
        n212 = Build Array (concatenate)(w392, w280) -> (w385:dbl[])
        n213 = Build Array (concatenate)(w391, w275) -> (w384:dbl[])
        n214 = Build Array (concatenate)(w471, w270) -> (w383:dbl[])
        n215 = Build Array (concatenate)(w343, w265) -> (w342:dbl[])
        n216 = Bundle(w389, w388, w387, w386, w385, w384, w383, w342, w345, w344) -> (w376:T10)  [unwired: 1 in]
        n217 = Unbundle(w376) -> (w294:dbl[], w252:dbl[], w291:dbl[], w282:dbl[], w277:dbl[], w272:dbl[], w267:dbl[], w261:dbl[], w257:dbl[], w251:dbl[])
        n218 = Bundle(w252, w294) -> (w295:cluster{dbl[], dbl[]})  [unwired: 1 in]
        n219 = Bundle(w252, w291) -> (w290:cluster{dbl[], dbl[]})  [unwired: 1 in]
        n220 = Bundle(w252, w282) -> (w281:cluster{dbl[], dbl[]})  [unwired: 1 in]
        n221 = Bundle(w252, w277) -> (w276:cluster{dbl[], dbl[]})  [unwired: 1 in]
        n222 = Bundle(w252, w267) -> (w266:cluster{dbl[], dbl[]})  [unwired: 1 in]
        n223 = Bundle(w252, w272) -> (w271:cluster{dbl[], dbl[]})  [unwired: 1 in]
        n224 = Bundle(w252, w261) -> (w262:cluster{dbl[], dbl[]})  [unwired: 1 in]
        n225 = Bundle(w252, w257) -> (w256:cluster{dbl[], dbl[]})  [unwired: 1 in]
        n226 = Bundle(w252, w251) -> (w250:cluster{dbl[], dbl[]})  [unwired: 1 in]
        n227 = Build Array(w295, w290, w281, w276, w271, w266, w262, w256, w250) -> (→"TIME GRAPH":cluster{dbl[], dbl[]}[])
        n228 = Unbundle(w376) -> (w375:dbl[], w374:dbl[], w373:dbl[], w372:dbl[], w371:dbl[], w370:dbl[], w369:dbl[], w368:dbl[], w337:dbl[])  [unwired: 1 out]
        n229 = case shown="\"V, Keithley DAQ A3\"" "X-Axis" {
          tunnel: [w501 w543 w578 w606 w648 w683 w718 w743 w778] -> w367
          tunnel: w375 -> [w498 w542 w577 w613 w647 w682 w716 w751 w786]
          tunnel: w374 -> [w515 w533 w576 w612 w646 w681 w715 w750 w785]
          tunnel: w373 -> [w514 w541 w568 w611 w645 w680 w714 w749 w784]
          tunnel: w372 -> [w513 w540 w575 w603 w644 w679 w713 w748 w783]
          tunnel: w371 -> [w512 w539 w574 w610 w638 w678 w712 w747 w782]
          tunnel: w370 -> [w511 w538 w573 w609 w643 w673 w711 w746 w781]
          tunnel: w369 -> [w510 w537 w572 w608 w642 w677 w717 w745 w780]
          tunnel: w368 -> [w509 w536 w571 w607 w641 w676 w710 w752 w779]
          tunnel: w337 -> [w499 w534 w569 w604 w639 w674 w709 w744 w787]
          frame "I, Keithley 6221", Default {
            n230 = Bundle(w498, w515) -> (w508:cluster{dbl[], dbl[]})  [unwired: 1 in]
            n231 = Bundle(w498, w514) -> (w507:cluster{dbl[], dbl[]})  [unwired: 1 in]
            n232 = Bundle(w498, w513) -> (w506:cluster{dbl[], dbl[]})  [unwired: 1 in]
            n233 = Bundle(w498, w512) -> (w505:cluster{dbl[], dbl[]})  [unwired: 1 in]
            n234 = Bundle(w498, w511) -> (w504:cluster{dbl[], dbl[]})  [unwired: 1 in]
            n235 = Bundle(w498, w510) -> (w503:cluster{dbl[], dbl[]})  [unwired: 1 in]
            n236 = Bundle(w498, w509) -> (w502:cluster{dbl[], dbl[]})  [unwired: 1 in]
            n237 = Bundle(w498, w499) -> (w500:cluster{dbl[], dbl[]})  [unwired: 1 in]
            n238 = Build Array(w508, w507, w506, w505, w504, w503, w502, w500) -> (w501:cluster{dbl[], dbl[]}[])
            n239 = property on="MULTIPLE GRAPHS" class="XYGraph (strict)"("XScale.NameLbl.Text"="Keithley 6221, mA" ("X Scale.Name Label.Text")) -> ()  [unwired: 2 in, 2 out]
            n240 = property on="MULTIPLE GRAPHS" class="XYGraph (strict)"("Active Plot"=u32 0, "Plot.Plot Name"="Mult, 2000 V", "Active Plot"=u32 1, "Plot.Plot Name"="DAQ A0", "Active Plot"=u32 2, "Plot.Plot Name"="DAQ A1", "Active Plot"=u32 3, "Plot.Plot Name"="DAQ A2", "Active Plot"=u32 4, "Plot.Plot Name"="DAQ A3", "Active Plot"=u32 5, "Plot.Plot Name"="DAQ A4", "Active Plot"=u32 6, "Plot.Plot Name"="Lock-In, X", "Active Plot"=u32 7, "Plot.Plot Name"="Lock-In, Y") -> ()  [unwired: 2 in, 2 out]
          }
          frame "V, Keithley 2000" {
            n241 = property on="MULTIPLE GRAPHS" class="XYGraph (strict)"("XScale.NameLbl.Text"="Keithley 2000, V" ("X Scale.Name Label.Text")) -> ()  [unwired: 2 in, 2 out]
            n242 = Bundle(w533, w542) -> (w550:cluster{dbl[], dbl[]})  [unwired: 1 in]
            n243 = Bundle(w533, w541) -> (w549:cluster{dbl[], dbl[]})  [unwired: 1 in]
            n244 = Bundle(w533, w540) -> (w548:cluster{dbl[], dbl[]})  [unwired: 1 in]
            n245 = Bundle(w533, w539) -> (w547:cluster{dbl[], dbl[]})  [unwired: 1 in]
            n246 = Bundle(w533, w538) -> (w546:cluster{dbl[], dbl[]})  [unwired: 1 in]
            n247 = Bundle(w533, w537) -> (w545:cluster{dbl[], dbl[]})  [unwired: 1 in]
            n248 = Bundle(w533, w536) -> (w544:cluster{dbl[], dbl[]})  [unwired: 1 in]
            n249 = Bundle(w533, w534) -> (w535:cluster{dbl[], dbl[]})  [unwired: 1 in]
            n250 = Build Array(w550, w549, w548, w547, w546, w545, w544, w535) -> (w543:cluster{dbl[], dbl[]}[])
            n251 = property on="MULTIPLE GRAPHS" class="XYGraph (strict)"("Active Plot"=u32 0, "Plot.Plot Name"="I, 6221 mA", "Active Plot"=u32 1, "Plot.Plot Name"="DAQ A0", "Active Plot"=u32 2, "Plot.Plot Name"="DAQ A1", "Active Plot"=u32 3, "Plot.Plot Name"="DAQ A2", "Active Plot"=u32 4, "Plot.Plot Name"="DAQ A3", "Active Plot"=u32 5, "Plot.Plot Name"="DAQ A4", "Active Plot"=u32 6, "Plot.Plot Name"="Lock-In, X", "Active Plot"=u32 7, "Plot.Plot Name"="Lock-In, Y") -> ()  [unwired: 2 in, 2 out]
          }
          frame "V, Keithley DAQ A0" {
            n252 = property on="MULTIPLE GRAPHS" class="XYGraph (strict)"("XScale.NameLbl.Text"="Keithley DAQ A0, V" ("X Scale.Name Label.Text")) -> ()  [unwired: 2 in, 2 out]
            n253 = Bundle(w568, w569) -> (w570:cluster{dbl[], dbl[]})  [unwired: 1 in]
            n254 = Bundle(w568, w577) -> (w585:cluster{dbl[], dbl[]})  [unwired: 1 in]
            n255 = Bundle(w568, w576) -> (w584:cluster{dbl[], dbl[]})  [unwired: 1 in]
            n256 = Bundle(w568, w575) -> (w583:cluster{dbl[], dbl[]})  [unwired: 1 in]
            n257 = Bundle(w568, w574) -> (w582:cluster{dbl[], dbl[]})  [unwired: 1 in]
            n258 = Bundle(w568, w573) -> (w581:cluster{dbl[], dbl[]})  [unwired: 1 in]
            n259 = Bundle(w568, w572) -> (w580:cluster{dbl[], dbl[]})  [unwired: 1 in]
            n260 = Bundle(w568, w571) -> (w579:cluster{dbl[], dbl[]})  [unwired: 1 in]
            n261 = Build Array(w585, w584, w583, w582, w581, w580, w579, w570) -> (w578:cluster{dbl[], dbl[]}[])
            n262 = property on="MULTIPLE GRAPHS" class="XYGraph (strict)"("Active Plot"=u32 0, "Plot.Plot Name"="I, 6221 mA", "Active Plot"=u32 1, "Plot.Plot Name"="Mult, 2000 V", "Active Plot"=u32 2, "Plot.Plot Name"="DAQ A1", "Active Plot"=u32 3, "Plot.Plot Name"="DAQ A2", "Active Plot"=u32 4, "Plot.Plot Name"="DAQ A3", "Active Plot"=u32 5, "Plot.Plot Name"="DAQ A4", "Active Plot"=u32 6, "Plot.Plot Name"="Lock-In, X", "Active Plot"=u32 7, "Plot.Plot Name"="Lock-In, Y") -> ()  [unwired: 2 in, 2 out]
          }
          frame "V, Keithley DAQ A1" {
            n263 = property on="MULTIPLE GRAPHS" class="XYGraph (strict)"("XScale.NameLbl.Text"="Keithley DAQ A1, V" ("X Scale.Name Label.Text")) -> ()  [unwired: 2 in, 2 out]
            n264 = Bundle(w603, w613) -> (w615:cluster{dbl[], dbl[]})  [unwired: 1 in]
            n265 = Bundle(w603, w612) -> (w616:cluster{dbl[], dbl[]})  [unwired: 1 in]
            n266 = Bundle(w603, w611) -> (w617:cluster{dbl[], dbl[]})  [unwired: 1 in]
            n267 = Bundle(w603, w610) -> (w618:cluster{dbl[], dbl[]})  [unwired: 1 in]
            n268 = Bundle(w603, w609) -> (w619:cluster{dbl[], dbl[]})  [unwired: 1 in]
            n269 = Bundle(w603, w608) -> (w620:cluster{dbl[], dbl[]})  [unwired: 1 in]
            n270 = Bundle(w603, w607) -> (w621:cluster{dbl[], dbl[]})  [unwired: 1 in]
            n271 = Bundle(w603, w604) -> (w605:cluster{dbl[], dbl[]})  [unwired: 1 in]
            n272 = Build Array(w615, w616, w617, w618, w619, w620, w621, w605) -> (w606:cluster{dbl[], dbl[]}[])
            n273 = property on="MULTIPLE GRAPHS" class="XYGraph (strict)"("Active Plot"=u32 0, "Plot.Plot Name"="I, 6221 mA", "Active Plot"=u32 1, "Plot.Plot Name"="Mult, 2000 V", "Active Plot"=u32 2, "Plot.Plot Name"="DAQ A0", "Active Plot"=u32 3, "Plot.Plot Name"="DAQ A2", "Active Plot"=u32 4, "Plot.Plot Name"="DAQ A3", "Active Plot"=u32 5, "Plot.Plot Name"="DAQ A4", "Active Plot"=u32 6, "Plot.Plot Name"="Lock-In, X", "Active Plot"=u32 7, "Plot.Plot Name"="Lock-In, Y") -> ()  [unwired: 2 in, 2 out]
          }
          frame "V, Keithley DAQ A2" {
            n274 = property on="MULTIPLE GRAPHS" class="XYGraph (strict)"("XScale.NameLbl.Text"="Keithley DAQ A2, V" ("X Scale.Name Label.Text")) -> ()  [unwired: 2 in, 2 out]
            n275 = Bundle(w638, w647) -> (w649:cluster{dbl[], dbl[]})  [unwired: 1 in]
            n276 = Bundle(w638, w646) -> (w650:cluster{dbl[], dbl[]})  [unwired: 1 in]
            n277 = Bundle(w638, w645) -> (w651:cluster{dbl[], dbl[]})  [unwired: 1 in]
            n278 = Bundle(w638, w644) -> (w652:cluster{dbl[], dbl[]})  [unwired: 1 in]
            n279 = Bundle(w638, w643) -> (w653:cluster{dbl[], dbl[]})  [unwired: 1 in]
            n280 = Bundle(w638, w642) -> (w654:cluster{dbl[], dbl[]})  [unwired: 1 in]
            n281 = Bundle(w638, w641) -> (w655:cluster{dbl[], dbl[]})  [unwired: 1 in]
            n282 = Bundle(w638, w639) -> (w640:cluster{dbl[], dbl[]})  [unwired: 1 in]
            n283 = Build Array(w649, w650, w651, w652, w653, w654, w655, w640) -> (w648:cluster{dbl[], dbl[]}[])
            n284 = property on="MULTIPLE GRAPHS" class="XYGraph (strict)"("Active Plot"=u32 0, "Plot.Plot Name"="I, 6221 mA", "Active Plot"=u32 1, "Plot.Plot Name"="Mult, 2000 V", "Active Plot"=u32 2, "Plot.Plot Name"="DAQ A0", "Active Plot"=u32 3, "Plot.Plot Name"="DAQ A1", "Active Plot"=u32 4, "Plot.Plot Name"="DAQ A3", "Active Plot"=u32 5, "Plot.Plot Name"="DAQ A4", "Active Plot"=u32 6, "Plot.Plot Name"="Lock-In, X", "Active Plot"=u32 7, "Plot.Plot Name"="Lock-In, Y") -> ()  [unwired: 2 in, 2 out]
          }
          frame "V, Keithley DAQ A3" {
            n285 = property on="MULTIPLE GRAPHS" class="XYGraph (strict)"("XScale.NameLbl.Text"="Keithley DAQ A3, V" ("X Scale.Name Label.Text")) -> ()  [unwired: 2 in, 2 out]
            n286 = Bundle(w673, w682) -> (w684:cluster{dbl[], dbl[]})  [unwired: 1 in]
            n287 = Bundle(w673, w681) -> (w685:cluster{dbl[], dbl[]})  [unwired: 1 in]
            n288 = Bundle(w673, w680) -> (w686:cluster{dbl[], dbl[]})  [unwired: 1 in]
            n289 = Bundle(w673, w679) -> (w687:cluster{dbl[], dbl[]})  [unwired: 1 in]
            n290 = Bundle(w673, w678) -> (w688:cluster{dbl[], dbl[]})  [unwired: 1 in]
            n291 = Bundle(w673, w677) -> (w689:cluster{dbl[], dbl[]})  [unwired: 1 in]
            n292 = Bundle(w673, w676) -> (w690:cluster{dbl[], dbl[]})  [unwired: 1 in]
            n293 = Bundle(w673, w674) -> (w675:cluster{dbl[], dbl[]})  [unwired: 1 in]
            n294 = Build Array(w684, w685, w686, w687, w688, w689, w690, w675) -> (w683:cluster{dbl[], dbl[]}[])
            n295 = property on="MULTIPLE GRAPHS" class="XYGraph (strict)"("Active Plot"=u32 0, "Plot.Plot Name"="I, 6221 mA", "Active Plot"=u32 1, "Plot.Plot Name"="Mult, 2000 V", "Active Plot"=u32 2, "Plot.Plot Name"="DAQ A0", "Active Plot"=u32 3, "Plot.Plot Name"="DAQ A1", "Active Plot"=u32 4, "Plot.Plot Name"="DAQ A2", "Active Plot"=u32 5, "Plot.Plot Name"="DAQ A4", "Active Plot"=u32 6, "Plot.Plot Name"="Lock-In, X", "Active Plot"=u32 7, "Plot.Plot Name"="Lock-In,Y") -> ()  [unwired: 2 in, 2 out]
          }
          frame "V, Keithley DAQ A4" {
            n296 = property on="MULTIPLE GRAPHS" class="XYGraph (strict)"("XScale.NameLbl.Text"="Keithley DAQ A4, V" ("X Scale.Name Label.Text")) -> ()  [unwired: 2 in, 2 out]
            n297 = Bundle(w717, w716) -> (w720:cluster{dbl[], dbl[]})  [unwired: 1 in]
            n298 = Bundle(w717, w715) -> (w721:cluster{dbl[], dbl[]})  [unwired: 1 in]
            n299 = Bundle(w717, w714) -> (w722:cluster{dbl[], dbl[]})  [unwired: 1 in]
            n300 = Bundle(w717, w713) -> (w723:cluster{dbl[], dbl[]})  [unwired: 1 in]
            n301 = Bundle(w717, w712) -> (w724:cluster{dbl[], dbl[]})  [unwired: 1 in]
            n302 = Bundle(w717, w711) -> (w725:cluster{dbl[], dbl[]})  [unwired: 1 in]
            n303 = Bundle(w717, w710) -> (w726:cluster{dbl[], dbl[]})  [unwired: 1 in]
            n304 = Bundle(w717, w709) -> (w719:cluster{dbl[], dbl[]})  [unwired: 1 in]
            n305 = Build Array(w720, w721, w722, w723, w724, w725, w726, w719) -> (w718:cluster{dbl[], dbl[]}[])
            n306 = property on="MULTIPLE GRAPHS" class="XYGraph (strict)"("Active Plot"=u32 0, "Plot.Plot Name"="I, 6221 mA", "Active Plot"=u32 1, "Plot.Plot Name"="Mult, 2000 V", "Active Plot"=u32 2, "Plot.Plot Name"="DAQ A0", "Active Plot"=u32 3, "Plot.Plot Name"="DAQ A1", "Active Plot"=u32 4, "Plot.Plot Name"="DAQ A2", "Active Plot"=u32 5, "Plot.Plot Name"="DAQ A3", "Active Plot"=u32 6, "Plot.Plot Name"="Lock-In, X", "Active Plot"=u32 7, "Plot.Plot Name"="Lock-In, Y") -> ()  [unwired: 2 in, 2 out]
          }
          frame "V, Lock-In X" {
            n307 = property on="MULTIPLE GRAPHS" class="XYGraph (strict)"("XScale.NameLbl.Text"="Lock-In X, V" ("X Scale.Name Label.Text")) -> ()  [unwired: 2 in, 2 out]
            n308 = Bundle(w752, w751) -> (w754:cluster{dbl[], dbl[]})  [unwired: 1 in]
            n309 = Bundle(w752, w750) -> (w755:cluster{dbl[], dbl[]})  [unwired: 1 in]
            n310 = Bundle(w752, w749) -> (w756:cluster{dbl[], dbl[]})  [unwired: 1 in]
            n311 = Bundle(w752, w748) -> (w757:cluster{dbl[], dbl[]})  [unwired: 1 in]
            n312 = Bundle(w752, w747) -> (w758:cluster{dbl[], dbl[]})  [unwired: 1 in]
            n313 = Bundle(w752, w746) -> (w759:cluster{dbl[], dbl[]})  [unwired: 1 in]
            n314 = Bundle(w752, w745) -> (w760:cluster{dbl[], dbl[]})  [unwired: 1 in]
            n315 = Bundle(w752, w744) -> (w753:cluster{dbl[], dbl[]})  [unwired: 1 in]
            n316 = Build Array(w754, w755, w756, w757, w758, w759, w760, w753) -> (w743:cluster{dbl[], dbl[]}[])
            n317 = property on="MULTIPLE GRAPHS" class="XYGraph (strict)"("Active Plot"=u32 0, "Plot.Plot Name"="I, 6221 mA", "Active Plot"=u32 1, "Plot.Plot Name"="Mult, 2000 V", "Active Plot"=u32 2, "Plot.Plot Name"="DAQ A0", "Active Plot"=u32 3, "Plot.Plot Name"="DAQ A1", "Active Plot"=u32 4, "Plot.Plot Name"="DAQ A2", "Active Plot"=u32 5, "Plot.Plot Name"="DAQ A3", "Active Plot"=u32 6, "Plot.Plot Name"="DAQ A4", "Active Plot"=u32 7, "Plot.Plot Name"="Lock-In, Y") -> ()  [unwired: 2 in, 2 out]
          }
          frame "V, Lock-In Y" {
            n318 = property on="MULTIPLE GRAPHS" class="XYGraph (strict)"("XScale.NameLbl.Text"="Lock-In Y, V" ("X Scale.Name Label.Text")) -> ()  [unwired: 2 in, 2 out]
            n319 = Bundle(w787, w786) -> (w795:cluster{dbl[], dbl[]})  [unwired: 1 in]
            n320 = Bundle(w787, w785) -> (w794:cluster{dbl[], dbl[]})  [unwired: 1 in]
            n321 = Bundle(w787, w784) -> (w793:cluster{dbl[], dbl[]})  [unwired: 1 in]
            n322 = Bundle(w787, w783) -> (w792:cluster{dbl[], dbl[]})  [unwired: 1 in]
            n323 = Bundle(w787, w782) -> (w791:cluster{dbl[], dbl[]})  [unwired: 1 in]
            n324 = Bundle(w787, w781) -> (w790:cluster{dbl[], dbl[]})  [unwired: 1 in]
            n325 = Bundle(w787, w780) -> (w789:cluster{dbl[], dbl[]})  [unwired: 1 in]
            n326 = Bundle(w787, w779) -> (w788:cluster{dbl[], dbl[]})  [unwired: 1 in]
            n327 = Build Array(w795, w794, w793, w792, w791, w790, w789, w788) -> (w778:cluster{dbl[], dbl[]}[])
            n328 = property on="MULTIPLE GRAPHS" class="XYGraph (strict)"("Active Plot"=u32 0, "Plot.Plot Name"="I, 6221 mA", "Active Plot"=u32 1, "Plot.Plot Name"="Mult, 2000 V", "Active Plot"=u32 2, "Plot.Plot Name"="DAQ A0", "Active Plot"=u32 3, "Plot.Plot Name"="DAQ A1", "Active Plot"=u32 4, "Plot.Plot Name"="DAQ A2", "Active Plot"=u32 5, "Plot.Plot Name"="DAQ A3", "Active Plot"=u32 6, "Plot.Plot Name"="DAQ A4", "Active Plot"=u32 7, "Plot.Plot Name"="Lock-In, X") -> ()  [unwired: 2 in, 2 out]
          }
        }
        "MULTIPLE GRAPHS" <- w367
        n329 = Unbundle(w376) -> (w382:dbl[], w381:dbl[], w380:dbl[], w379:dbl[], w378:dbl[], w377:dbl[], w338:dbl[], w339:dbl[], w340:dbl[], w341:dbl[])
        n330 = Multiply(x="Time Delay", y=u16 1000) -> (x*y=w242:u16)
        n331 = Wait Until Next ms Multiple(millisecond multiple=w242) -> ()  [unwired: 1 out]
        "2000" <- w464
        "DAQ A0" <- w351
        "DAQ A1" <- w350
        "DAQ A2" <- w349
        "DAQ A3" <- w348
        "DAQ A4" <- w347
      }
    }
    frame #3 {
      # "Closing instrumental \nconnections"
      n332 = Unbundle(w1120) -> ("Task out"=w1119:i32, "error out"=w1118:errorcluster)
      n333 = call <instrlib>:"Close.vi"("VISA resource name"=w1125, "error in (no error)"=w1126) -> ()  [unwired: 17 in, 1 out]
      n334 = call "SR51XX Close"("error in (no error)"=w1121, "VISA session"=w1122) -> ()  [unwired: 1 out]
      n335 = call <instrlib>:"Close.vi"("VISA resource name"=w1123, "error in (no error)"=w1124) -> ()  [unwired: 13 in, 1 out]
      n336 = call <userlib>:"DtOLCloseTask.vi"("Error in"=w1118, "Task in"=w1119) -> ("Error Out"=w1127:errorcluster)  [unwired: 9 in]
      n337 = call <vilib>:"Simple Error Handler.vi"("error in (no error)"=w1127) -> ()  [unwired: 4 in, 5 out]
    }
  }
